vi "Plots_testing_2.vi"() -> ()   [LabVIEW 2018]
panel:
  out "ms to show":dbl
  out "Waveform Chart 2":waveform(dbl)(graph)
  out "Waveform Chart":waveform(dbl)(graph)
  out "Waveform Chart - Light":waveform(dbl)(graph)
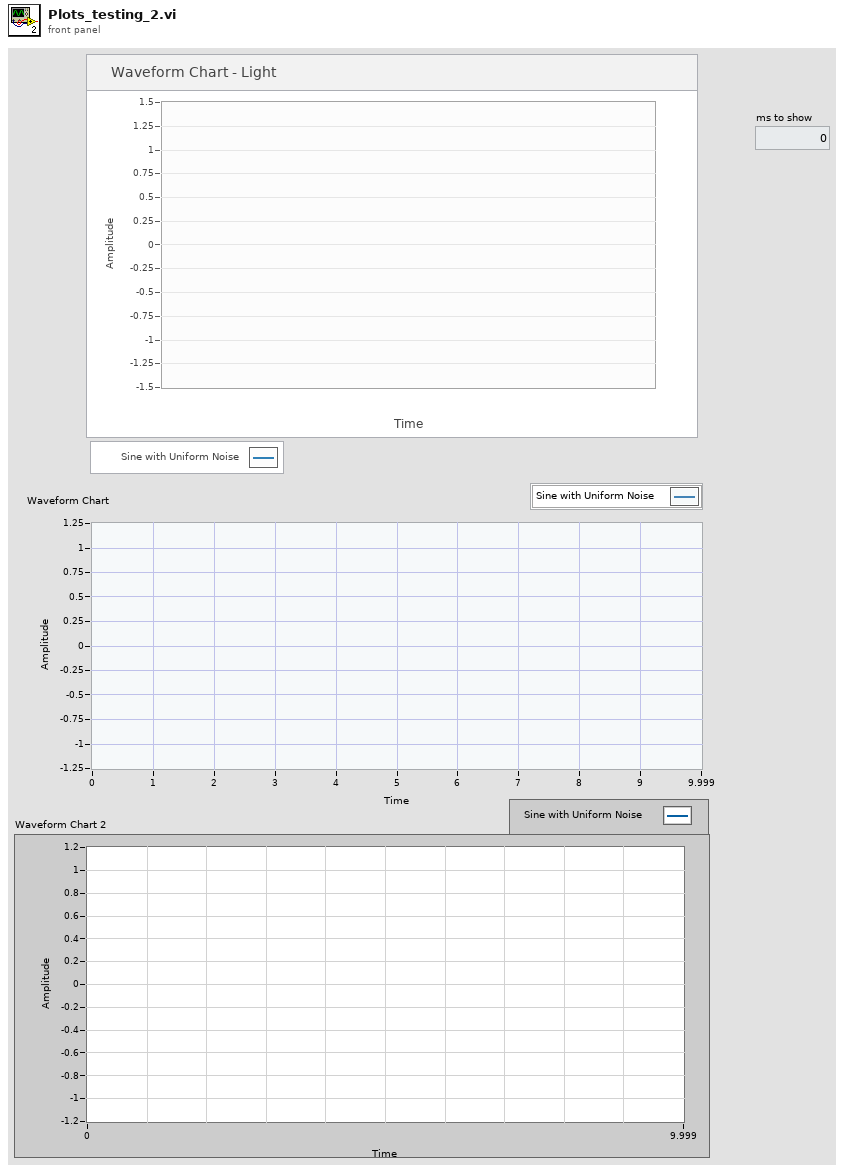
[diagram p1: front panel]
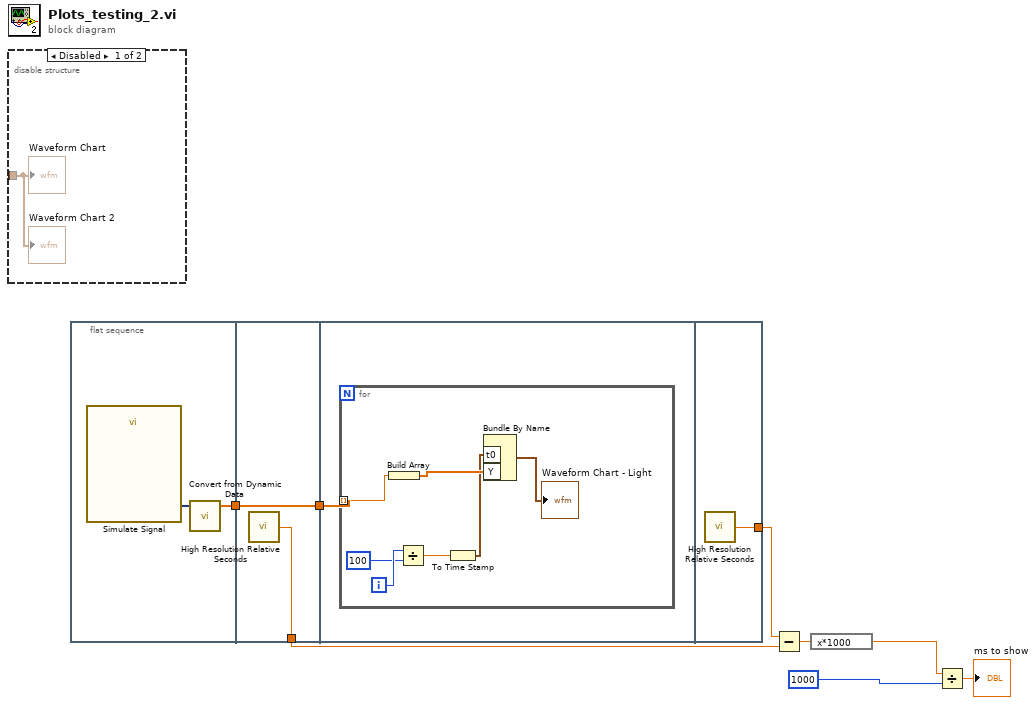
[diagram p0: block diagram]
diagram:
  n1 = disable-structure shown="Disabled" {
    disable-tunnel: _ -> [w9 _]
    frame Disabled {
      "Waveform Chart" <- w9
      "Waveform Chart 2" <- w9
    }
    frame Enabled {
    }
  }
  n2 = flat-sequence {
    tunnel: [w11] -> w6
    tunnel: [w13] -> w3
    tunnel: [w12] -> w5
    tunnel: w6 -> [w12]
    tunnel: w5 -> [w14]
    tunnel: [w22] -> w4
    frame #0 {
      n3 = call "Simulate Signal"() -> ("Sine with Gaussian Noise"=w10:dynamicdata)  [unwired: 14 in, 1 out]
      n4 = call "Convert from Dynamic Data"("Dynamic Data Type"=w10) -> ("Array"=w11:dbl[])  [unwired: 3 in]
    }
    frame #1 {
      n5 = call <vilib>:"High Resolution Relative Seconds.vi"() -> ("relative seconds"=w13:dbl)
    }
    frame #2 {
      n6 = for {
        tunnel: w14 -> [w20] mode=indexing
        i -> [w18]
        n7 = Build Array(w20) -> (w21:dbl[])
        n8 = Divide(x=w18, y=100) -> (x/y=w16:dbl)
        n9 = To Time Stamp(1:w16) -> (0:w15:timestamp)
        n10 = Bundle By Name("t0"=w15, "Y"=w21) -> (→"Waveform Chart - Light":waveform(dbl))  [unwired: 1 in]
      }
    }
    frame #3 {
      n11 = call <vilib>:"High Resolution Relative Seconds.vi"() -> ("relative seconds"=w22:dbl)
    }
  }
  n12 = Subtract(x=w4, y=w3) -> (x-y=w2:dbl)
  n13 = expression code="x*1000"(w2) -> (w1:dbl)
  n14 = Divide(x=w1, y=1000) -> (x/y=→"ms to show":dbl)
